vi "Create TCP Slave.vi"(4 "write operation timeout":i32=5000, 6 "read operation timeout":i32=5000, 8 "error in":errorcluster, 10 "port (502)":u16=502) -> (0 "error out":errorcluster, 3 "TCP slave instance":refnum<class "Modbus Slave.lvclass">)   [LabVIEW 2021, in "API Main.lvlib"]
doc: "Creates a standard TCP slave with an IP ADU. If the data model input is unwired, a standard data model will be initialized and used. If the input is wired, the code will check to make sure that it is not the default value for the class (it should be initialized). If the default value of the class is wired, the standard model will be initialized and used."
uses:
  API Main.lvlib
  Slave/Modbus Slave.lvclass
  Data Model/Device Data Model.lvclass
  Network Protocol/Network Slave/TCP/TCP Slave.lvclass
  D:/my_projects/projects/Algorithms/Labview/21/Modbus_v121c/Network Protocol/Network Slave/Network Slave.lvclass
  Transmission Data Unit/IP/IP Data Unit.lvclass
  D:/my_projects/projects/Algorithms/Labview/21/Modbus_v121c/Transmission Data Unit/Transmission Data Unit.lvclass
  Data Model/Standard Data Model/Standard Data Model.lvclass
  D:/my_projects/projects/Algorithms/Labview/21/Modbus_v121c/Data Model/Device Data Model.lvclass
  Transmission Data Unit/IP/IP Data Unit.lvclass/IP Data Unit.ctl
  Transmission Data Unit/Transmission Data Unit.lvclass/Transmission Data Unit.ctl
  Network Protocol/Network Slave/Network Slave.lvclass/Network Slave.ctl
  Slave/Modbus Slave.lvclass/Modbus Slave.ctl
  Data Model/Device Data Model.lvclass/Device Data Model.ctl
  Transmission Data Unit/IP/Write port.vi
  Transmission Data Unit/IP/Write connect timeout.vi
  Data Model/Read Initialized.vi
  <vilib>/Utility/error.llb/Clear Errors.vi
  Transmission Data Unit/Transmission Data Unit.lvclass
  Network Protocol/Network Slave/Network Slave.lvclass
panel:
  in  "connect timeout":i32=150000
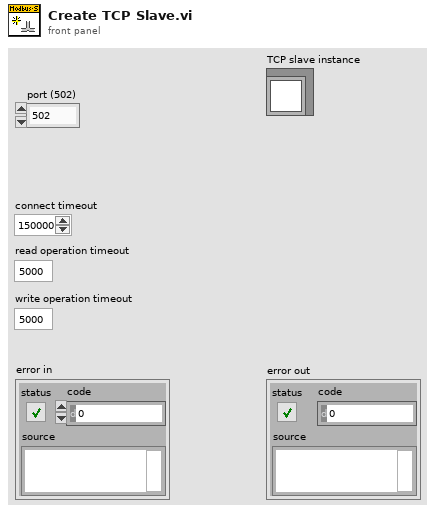
[diagram p1: front panel]
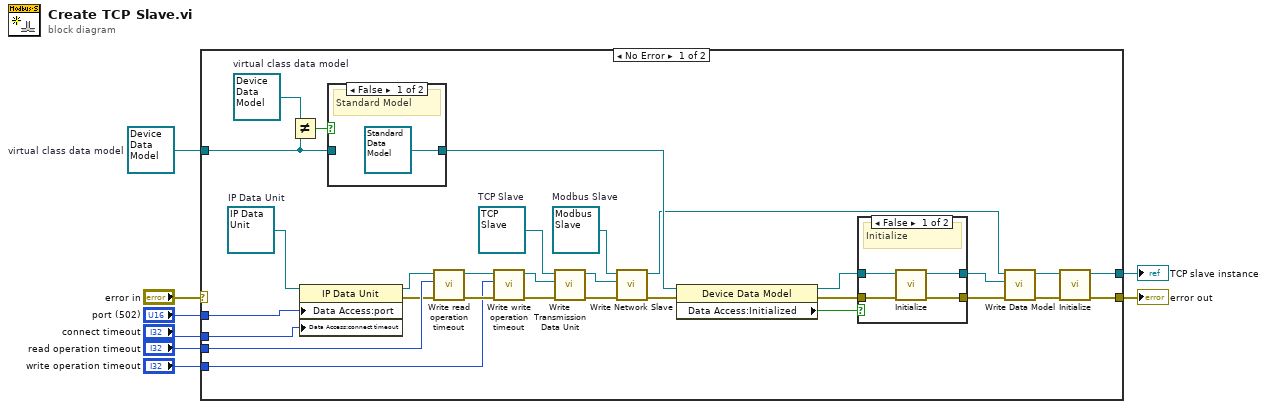
[diagram p0: block diagram]
diagram:
  w4 = refnum<class "Device Data Model.lvclass"> refnum  # virtual class data model
  n1 = case shown="No Error" "error in" {
    selector: "error in" -> [_ w47]
    tunnel: "port (502)" -> [w38 _]
    tunnel: [w37 w47] -> w2
    tunnel: [w36 _] -> w3
    tunnel: w4 -> [w30 _]
    tunnel: "write operation timeout" -> [w24 _]
    tunnel: "read operation timeout" -> [w23 _]
    tunnel: "connect timeout" -> [w9 _]
    frame No Error {
      w22 = refnum<class "IP Data Unit.lvclass"> refnum  # IP Data Unit
      w32 = refnum<class "Device Data Model.lvclass"> refnum  # virtual class data model
      w21 = refnum<class "TCP Slave.lvclass"> refnum  # TCP Slave
      w17 = refnum<class "Modbus Slave.lvclass"> refnum  # Modbus Slave
      n2 = Not Equal?(x=w32, y=w30) -> (x != y?=w31:bool)
      n3 = property class="IP Data Unit"(reference=w22, "Data Access:port"=w38, "Data Access:connect timeout"=w9) -> (reference out=w10:refnum<class "IP Data Unit.lvclass">, error out=w11:errorcluster)  [unwired: 1 in]
      n4 = case shown="False" w31 {
        tunnel: w30 -> [_ w40]
        tunnel: [refnum<class "Standard Data Model.lvclass"> refnum ("Standard Data Model") w40] -> w29
        frame False {
          # "Standard Model"
        }
        frame True {
        }
      }
      n5 = call "Write read operation timeout.vi"("error in (no error)"=w11, "read operation timeout"=w23, "transmission data unit in"=w10) -> ("error out"=w26:errorcluster, "transmission data unit out"=w25:refnum<class "IP Data Unit.lvclass">)  [unwired: 7 in]
      n6 = call "Write write operation timeout.vi"("error in (no error)"=w26, "write operation timeout"=w24, "transmission data unit in"=w25) -> ("error out"=w13:errorcluster, "transmission data unit out"=w12:refnum<class "IP Data Unit.lvclass">)  [unwired: 7 in]
      n7 = call "Write Transmission Data Unit.vi"("error in (no error)"=w13, "Transmission Data Unit"=w12, "Network Slave in"=w21) -> ("error out"=w20:errorcluster, "Network Slave out"=w19:refnum<class "TCP Slave.lvclass">)  [unwired: 7 in]
      n8 = call "Write Network Slave.vi"("error in (no error)"=w20, "Network Slave"=w19, "Modbus Slave in"=w17) -> ("error out"=w18:errorcluster, "Modbus Slave out"=w16:refnum<class "Modbus Slave.lvclass">)  [unwired: 7 in]
      n9 = property class="Device Data Model"(reference=w29, error in=w18) -> (reference out=w34:refnum<class "Device Data Model.lvclass">, error out=w35:errorcluster, "Data Access:Initialized"=w33:bool)
      n10 = case shown="False" w33 {
        tunnel: w35 -> [w44 w46]
        tunnel: [w43 w46] -> w27
        tunnel: [w42 w45] -> w28
        tunnel: w34 -> [w41 w45]
        frame False {
          # "Initialize"
          n11 = call-dynamic "Initialize.vi"("error in"=w44, "device data model in"=w41) -> ("error out"=w43:errorcluster, "device data model out"=w42:refnum<class "Device Data Model.lvclass">)  [unwired: 8 in]
        }
        frame True {
        }
      }
      n12 = call "Write Data Model.vi"("error in (no error)"=w27, "device data model"=w28, "Modbus slave in"=w16) -> ("error out"=w15:errorcluster, "Modbus slave out"=w14:refnum<class "Modbus Slave.lvclass">)  [unwired: 7 in]
      n13 = call-dynamic "Initialize.vi"("error in (no error)"=w15, "Modbus slave in"=w14) -> ("error out"=w37:errorcluster, "Modbus slave out"=w36:refnum<class "Modbus Slave.lvclass">)  [unwired: 8 in]
    }
    frame Error {
    }
  }
  "error out" <- w2
  "TCP slave instance" <- w3
